vi "GetTerms.vi"(0 "XRef":T12, 1 "State In":T10) -> (14 "Terms":T2, 15 "Fatal Error Out":T1)   [LabVIEW 2021, in "myRIO AI Open.xnode"]
uses:
  <vilib>/myRIO/Instrument Drivers/Onboard IO/AI/vis/myRIO AI Open.xnode
  <vilib>/XNodeSupport/XNodeXNodeRef.ctl
  <vilib>/myRIO/Instrument Drivers/Onboard IO/AI/vis/State.ctl
  <vilib>/myRIO/Common/Instrument Driver Framework/Utilities/typedefs/myRIOXPeripheral.ctl
  <vilib>/XNodeSupport/XNodeTerm4Array.ctl
  <vilib>/XNodeSupport/XNodeTerm4.ctl
  <vilib>/XNodeSupport/XNodeString.ctl
  <vilib>/XNodeSupport/XNodeVariant.ctl
  <vilib>/XNodeSupport/XNodeRect32.ctl
  <vilib>/XNodeSupport/XNodeInt.ctl
  <vilib>/XNodeSupport/XNodeBool.ctl
  <vilib>/XNodeSupport/XNodeTermDirection.ctl
  <vilib>/XNodeSupport/XNodeErrorCluster.ctl
  <vilib>/myRIO/Common/Instrument Driver Framework/Utilities/vis/myRIOXGlobal.vi
  <vilib>/myRIO/Common/FPGA Personality Framework/Personality.lvlib
  <vilib>/XNodeSupport/NI_XNodeSupport.lvlib
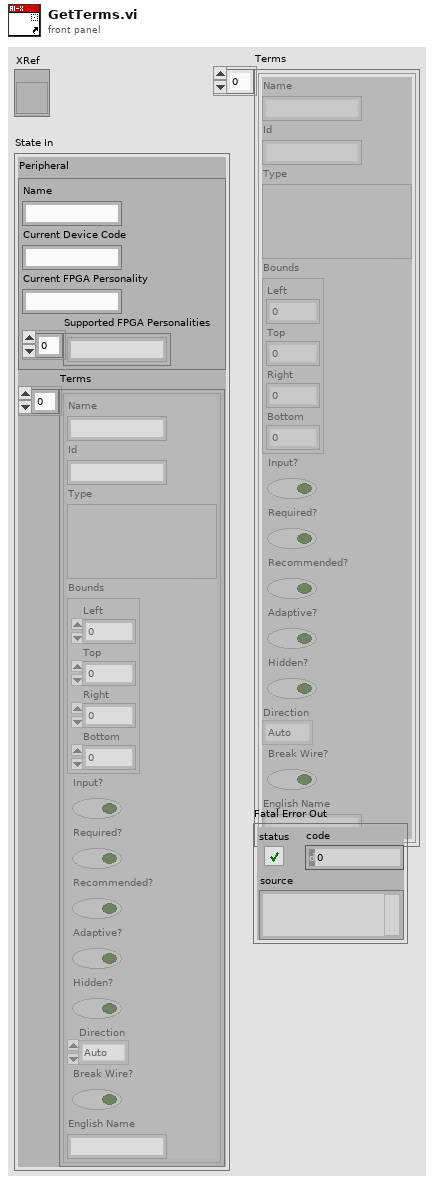
[diagram p1: front panel]
types:
  T1 = typedef "NI_XNodeSupport.lvlib/XNodeErrorCluster.ctl" = errorcluster
  T2 = typedef "NI_XNodeSupport.lvlib/XNodeTerm4Array.ctl" = T3[]
  T3 = typedef "NI_XNodeSupport.lvlib/XNodeTerm4.ctl" = cluster{"Name":T4, "Id":T4, "Type":T5, "Bounds":T6, "Input?":T8, "Required?":T8, "Recommended?":T8, "Adaptive?":T8, "Hidden?":T8, "Direction":T9, "Break Wire?":T8, "English Name":T4}
  T4 = typedef "NI_XNodeSupport.lvlib/XNodeString.ctl" = string
  T5 = typedef "NI_XNodeSupport.lvlib/XNodeVariant.ctl" = variant
  T6 = typedef "NI_XNodeSupport.lvlib/XNodeRect32.ctl" = cluster{"Left":T7, "Top":T7, "Right":T7, "Bottom":T7}
  T7 = typedef "NI_XNodeSupport.lvlib/XNodeInt.ctl" = i32
  T8 = typedef "NI_XNodeSupport.lvlib/XNodeBool.ctl" = bool
  T9 = typedef "NI_XNodeSupport.lvlib/XNodeTermDirection.ctl" = enum32{"Auto", "Up", "Down", "Left", "Right", "Center"}
  T10 = typedef "myRIO AI Open.xnode/State.ctl" = cluster{"Peripheral":T11, "Terms":T2}
  T11 = typedef "myRIOXPeripheral.ctl" = cluster{"Name":string, "Current Device Code":string, "Current FPGA Personality":string, "Supported FPGA Personalities":string[]}
  T12 = typedef "NI_XNodeSupport.lvlib/XNodeXNodeRef.ctl" = refnum<vi>
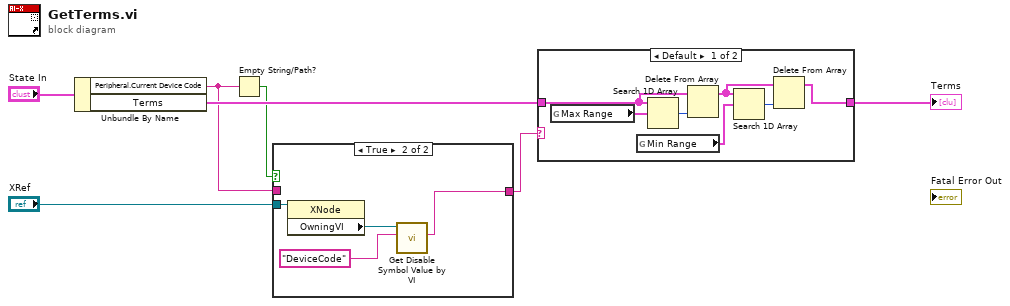
[diagram p0: block diagram]
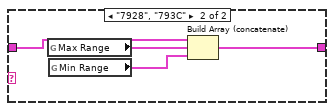
[diagram p3: hidden frame]
diagram:
  n1 = Unbundle By Name("State In") -> ("Peripheral.Current Device Code"=w2:string, "Terms"=w5:T2)
  n2 = Empty String/Path?(string/path=w2) -> (empty?=w3:bool)
  n3 = case shown="True" w3 {
    tunnel: "XRef" -> [_ w11]
    tunnel: [w8 w9] -> w1
    tunnel: w2 -> [w8 _]
    frame False {
    }
    frame True {
      n4 = property class="XNode"(reference=w11) -> ("OwningVI"=w10:refnum<vi>)  [unwired: 1 in, 2 out]
      n5 = call <vilib>:"Get Disable Symbol Value by VI.vi"("Disable Symbol"="DeviceCode", "VI Refnum"=w10) -> ("Value"=w9:string)  [unwired: 7 in, 2 out]
    }
  }
  n6 = case shown="Default" w1 {
    tunnel: [w13 w23] -> w6
    tunnel: w5 -> [w17 w20]
    frame Default {
      n7 = global read "myRIOXGlobal.vi" "Max Range"() -> (w19:T3)
      n8 = global read "myRIOXGlobal.vi" "Min Range"() -> (w15:T3)
      n9 = Search 1D Array(1D array=w17, element=w19) -> (index of element=w18:i32)  [unwired: 1 in]
      n10 = Delete From Array(array=w17, index=w18) -> (array with subset deleted=w14:T2)  [unwired: 1 in, 1 out]
      n11 = Search 1D Array(1D array=w14, element=w15) -> (index of element=w16:i32)  [unwired: 1 in]
      n12 = Delete From Array(array=w14, index=w16) -> (array with subset deleted=w13:T2)  [unwired: 1 in, 1 out]
    }
    frame "7928", "793C" {
      n13 = global read "myRIOXGlobal.vi" "Max Range"() -> (w22:T3)
      n14 = global read "myRIOXGlobal.vi" "Min Range"() -> (w21:T3)
      n15 = Build Array (concatenate)(w20, w22, w21) -> (w23:T2)
    }
  }
  "Terms" <- w6
